vi "JSONRPC-Error.vi"(8 "error in":errorcluster, 11 "Type":T1(ring)) -> (0 "error out":errorcluster)   [LabVIEW 2020]
doc: "Convert a JSON string into an array of elements."
panel:
  # "BuildResponse"
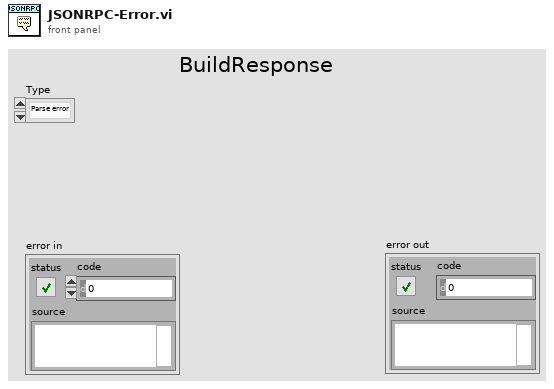
[diagram p1: front panel]
types:
  T1 = enum16{"Parse error", "Invalid request", "Method not found", "Invalid params", "Internal error", "Server error", ""}
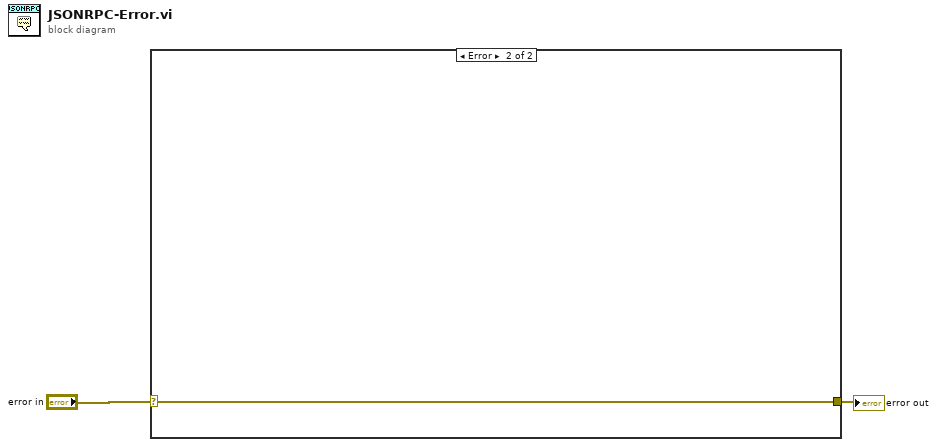
[diagram p0: block diagram]
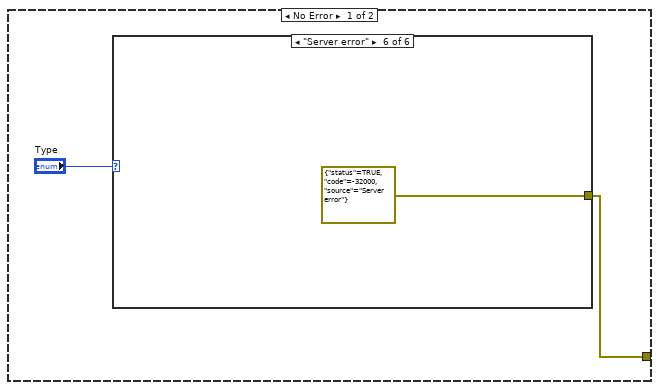
[diagram p2: hidden frame]
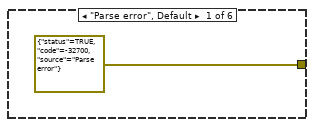
[diagram p3: hidden frame]
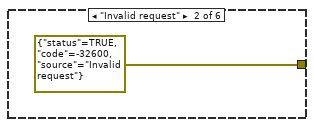
[diagram p4: hidden frame]
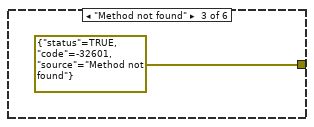
[diagram p5: hidden frame]
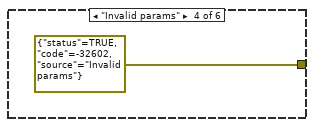
[diagram p6: hidden frame]
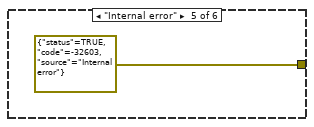
[diagram p7: hidden frame]
diagram:
  n1 = case shown="Error" "error in" {
    selector: "error in" -> [_ w11]
    tunnel: [w3 w11] -> w1
    frame No Error {
      n2 = case shown="\"Server error\"" "Type" {
        tunnel: [errorcluster {"status"=TRUE, "code"=-32700, "source"="Parse error"} ("error in 2") errorcluster {"status"=TRUE, "code"=-32600, "source"="Invalid request"} ("error in 2") errorcluster {"status"=TRUE, "code"=-32601, "source"="Method not found"} ("error in 2") errorcluster {"status"=TRUE, "code"=-32602, "source"="Invalid params"} ("error in 2") errorcluster {"status"=TRUE, "code"=-32603, "source"="Internal error"} ("error in 2") errorcluster {"status"=TRUE, "code"=-32000, "source"="Server error"} ("error in 2")] -> w3
        frame "Parse error", Default {
        }
        frame "Invalid request" {
        }
        frame "Method not found" {
        }
        frame "Invalid params" {
        }
        frame "Internal error" {
        }
        frame "Server error" {
        }
      }
    }
    frame Error {
    }
  }
  "error out" <- w1
